vi "Dyn - State To Execute.vi"(0 "LVx - Connect Instrument Command in":refnum<class "Rex - NART - Transmit.lvclass">, 11 "error in (no error)":errorcluster) -> (4 "LVx - Connect Instrument Command out":refnum<class "Rex - NART - Transmit.lvclass">, 8 "State To Execute":string, 15 "error out":errorcluster)   [LabVIEW 2011, in "ART2 Test Panel.lvlib" / "Rex - NART - Transmit.lvclass"]
uses:
  Rex - NART - Transmit.lvclass
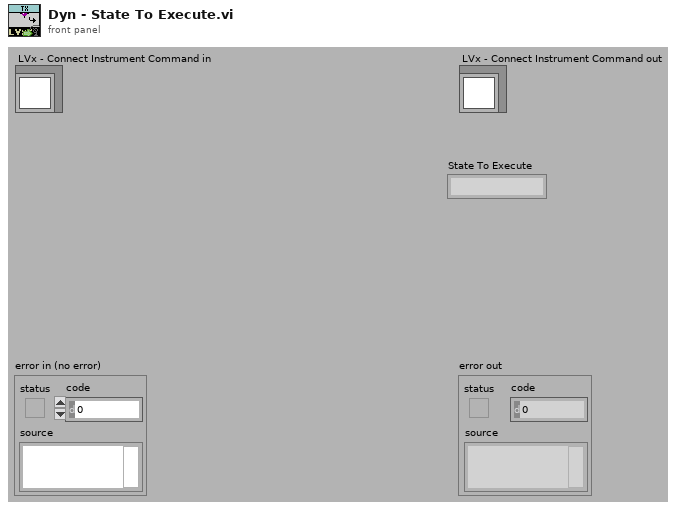
[diagram p1: front panel]
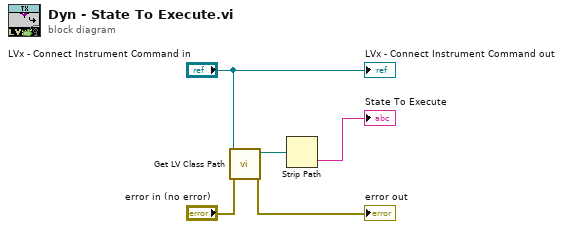
[diagram p0: block diagram]
diagram:
  n1 = call <vilib>:"Get LV Class Path.vi"("error in (no error)"="error in (no error)", "object"="LVx - Connect Instrument Command in") -> ("error out"=→"error out":errorcluster, "class path"=w4:path)  [unwired: 8 in]
  n2 = Strip Path(path=w4) -> (name=→"State To Execute":string)  [unwired: 1 out]
  "LVx - Connect Instrument Command out" <- "LVx - Connect Instrument Command in"
